vi "Entry.vi"(8 "error in (no error)":errorcluster, 11 "New State":refnum<class "Connected.lvclass">) -> (0 "error out":errorcluster, 3 "State out":refnum<class "Connected.lvclass">)   [LabVIEW 2013, in "Receiver.lvlib" / "Receiver Commands Using Processor.lvlib" / "Connect Command.lvlib" / "Connected.lvclass"]
doc: "This is an abstract method. Override this method to define the behavior when you enter the state."
uses:
  Connected.lvclass
  Connect Command.lvclass
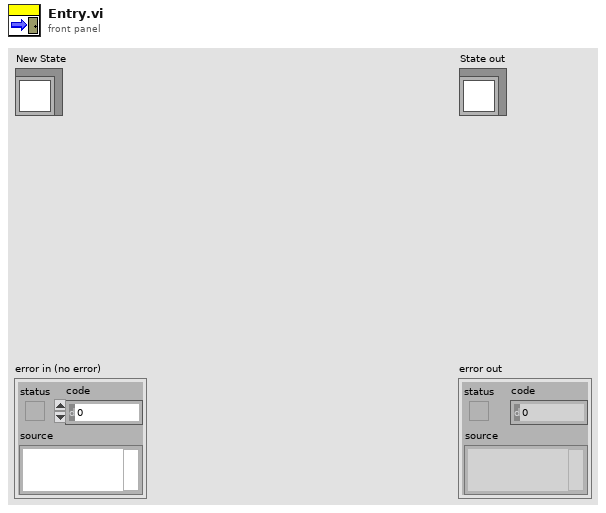
[diagram p1: front panel]
types:
  T1 = typedef "Command Processor.lvlib/Command.lvlib/Command.lvclass/Command Status.ctl" = cluster{"Command Name":string, "Current State Status":T2, "Command Start Time":timestamp, "Command End Time":timestamp, "Previous State Status":T2}
  T2 = typedef "Command Processor.lvlib/Command.lvlib/Command.lvclass/State Status.ctl" = cluster{"State Name":string, "State Entry Time":timestamp, "State Exit Time":timestamp}
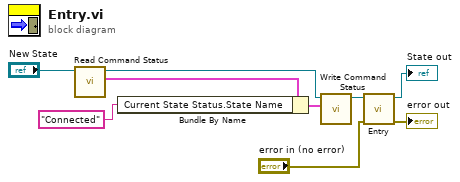
[diagram p0: block diagram]
diagram:
  n1 = call-dynamic "Read Command Status.vi"("Command in"="New State") -> ("Command Status"=w3:T1, "Command out"=w4:refnum<class "Connected.lvclass">)  [unwired: 8 in, 1 out]
  n2 = Bundle By Name(cluster=w3, "Current State Status.State Name"="Connected") -> (w2:T1)
  n3 = call-dynamic "Write Command Status.vi"("Command Status"=w2, "Command in"=w4) -> ("Command out"=w5:refnum<class "Connected.lvclass">)  [unwired: 8 in, 1 out]
  n4 = call-parent "Entry.vi"("error in (no error)"="error in (no error)", "New State"=w5) -> ("error out"=→"error out":errorcluster, "State out"=→"State out":refnum<class "Connected.lvclass">)  [unwired: 8 in]
